vi "Apply_19V_to_VBAT.vi"(3 "error in":errorcluster) -> (10 "error out":errorcluster)   [LabVIEW 2015]
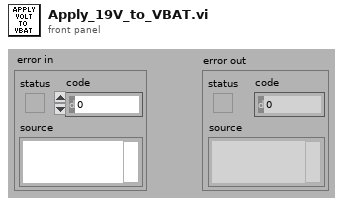
[diagram p1: front panel]
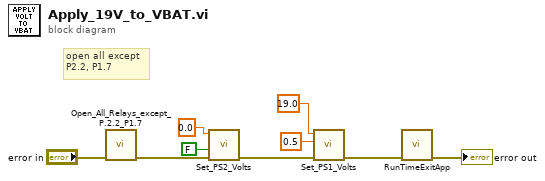
[diagram p0: block diagram]
diagram:
  # "open all except \nP2.2, P1.7"
  n1 = call "Open_All_Relays_except_P.2.2_P1.7.vi"("error in"="error in") -> ("error out"=w2:errorcluster)  [unwired: 8 in]
  n2 = call "Set_PS2_Volts.vi"("error in"=w2, "Output on/off"=FALSE, "Output Voltage"=0.0) -> ("error out"=w1:errorcluster)  [unwired: 6 in, 2 out]
  n3 = call "Set_PS1_Volts.vi"("error in"=w1, "delay (secs)"=0.5, "Output Voltage"=19.0) -> ("error out"=w5:errorcluster)  [unwired: 6 in, 2 out]
  n4 = call "RunTimeExitApp.vi"("error in (no error)"=w5) -> ("error out"=→"error out":errorcluster)  [unwired: 10 in]
